vi "Read VNA ports.vi"(11 "S Parameter in":refnum<class "S Parameter.lvclass">) -> (2 "VNA ports":bool[](array[boolean])=[TRUE, FALSE, FALSE, FALSE], 3 "S Parameter out":refnum<class "S Parameter.lvclass">)   [LabVIEW 2020, in "S Parameter.lvclass"]
uses:
  S Parameter.lvclass
  S Parameter.lvclass/S Parameter.ctl
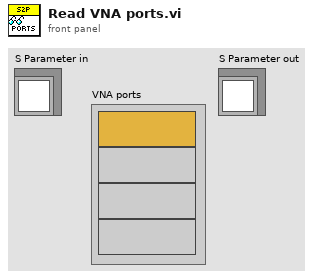
[diagram p1: front panel]
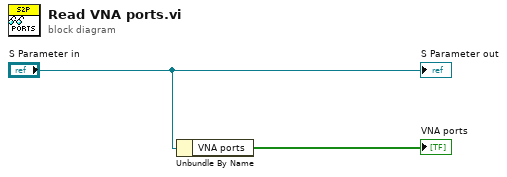
[diagram p0: block diagram]
diagram:
  n1 = Unbundle By Name("S Parameter in") -> ("VNA ports"=→"VNA ports":bool[])
  "S Parameter out" <- "S Parameter in"
